vi "RTD_try_open.vi"(8 "error in":errorcluster, 11 "thermo in":T1={"type"=enum."COMET Tx5xx (ethernet)", "comment"="", "tag"="", "refresh"=0.0, "IP"="", "port"=0, "VISA"="", "last readout"=timestamp(0 s since 1904-01-01), "TCP ref"=refnum, "VISA sess"="", "idn"="", "press"=0.0, "RH"=0.0, "temp"=0.0, "pres cor"=[], "RH cor"=[], "temp cor"=[], "try left"=0, "failed"=FALSE, "RTD set"=[], "RTD inv"=[], "range"=0.0, "net mode"=enum."MODBUS", "try fail"=enum."Stop trying - return NaN", "timeout [s]"=0.0, "max retries"=0, "sim t [deg]"=0.0, "status"=0} {"status" items=["ok", "retry", "failed"]; "RTD inv" format="%.1f"; "RTD set" format="%.1f"; "temp cor" format="%.1f"; "RH cor" format="%.1f"; "pres cor" format="%.1f"; "refresh" min=0.1 max=1000.0 format="%.2f"}) -> (0 "error out":errorcluster, 3 "thermo out":T1={"type"=enum."COMET Tx5xx (ethernet)", "comment"="", "tag"="", "refresh"=5.0, "IP"="", "port"=502, "VISA"="", "last readout"=timestamp(0 s since 1904-01-01), "TCP ref"=refnum, "VISA sess"="", "idn"="", "press"=0.0, "RH"=0.0, "temp"=0.0, "pres cor"=[], "RH cor"=[], "temp cor"=[], "try left"=0, "failed"=FALSE, "RTD set"=[], "RTD inv"=[], "range"=0.0, "net mode"=enum."MODBUS", "try fail"=enum."Stop trying - return NaN", "timeout [s]"=0.0, "max retries"=0, "sim t [deg]"=0.0, "status"=0} {"status" items=["ok", "retry", "failed"]; "RTD inv" format="%.1f"; "RTD set" format="%.1f"; "temp cor" format="%.1f"; "RH cor" format="%.1f"; "pres cor" format="%.1f"; "refresh" min=0.1 max=1000.0 format="%.2f"})   [LabVIEW 2020]
uses:
  thermo.ctl
  thermo_types.ctl
  Thermometer Fail Action.ctl
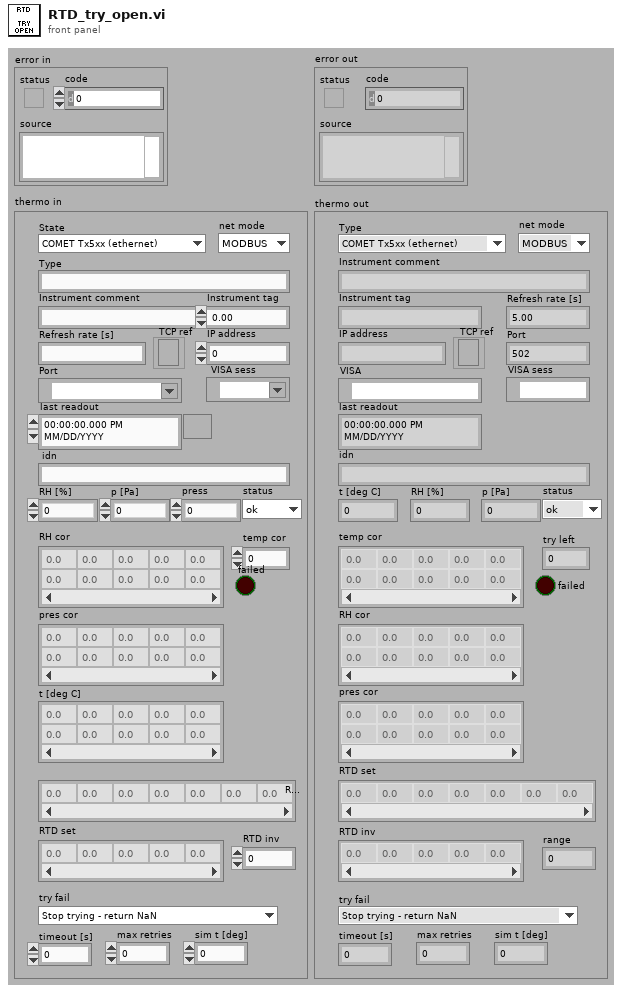
[diagram p1: front panel]
types:
  T1 = typedef "thermo.ctl" = cluster{"type":T2, "comment":string, "tag":string, "refresh":dbl, "IP":string, "port":u16, "VISA":refnum<visa-resource-name>, "last readout":timestamp, "TCP ref":refnum<k5>, "VISA sess":refnum<visa-resource-name>, "idn":string, "press":dbl, "RH":dbl, "temp":dbl, "pres cor":dbl[][], "RH cor":dbl[][], "temp cor":dbl[][], "try left":i32, "failed":bool, "RTD set":dbl[], "RTD inv":dbl[], "range":dbl, "net mode":enum16{"MODBUS", "HTTP"}, "try fail":T3, "timeout [s]":dbl, "max retries":i32, "sim t [deg]":dbl, "status":u16}
  T2 = typedef "thermo_types.ctl" = enum16{"Disabled", "Simulated", "COMET Tx5xx (ethernet)", "Keithley 2002 (GPIB) + RTD", "Agilent 344xx (GPIB) + RTD"}
  T3 = typedef "Thermometer Fail Action.ctl" = enum16{"Stop trying - keep last value", "Stop trying - return NaN", "Generate error - stop sweep"}
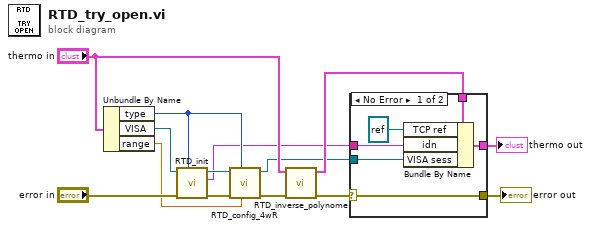
[diagram p0: block diagram]
diagram:
  n1 = Unbundle By Name("thermo in") -> ("type"=w9:T2, "VISA"=w10:refnum<visa-resource-name>, "range"=w8:dbl)
  n2 = call "RTD_init.vi"("type"=w9, "error in"="error in", "VISA in"=w10) -> ("error out"=w14:errorcluster, "ID"=w5:string, "VISA out"=w13:refnum<visa-resource-name>)  [unwired: 6 in]
  n3 = call "RTD_config_4wR.vi"("range [Ohm]"=w8, "type"=w9, "error in"=w14, "VISA in"=w13) -> ("error out"=w12:errorcluster, "VISA out"=w4:refnum<visa-resource-name>)  [unwired: 6 in]
  n4 = call "RTD_inverse_polynome.vi"("error in"=w12, "channel in"="thermo in") -> ("error out"=w3:errorcluster, "channel out"=w6:T1)  [unwired: 8 in]
  n5 = case shown="No Error" w3 {
    selector: w3 -> [w16 w22]
    tunnel: w6 -> [w20 w21]
    tunnel: w5 -> [w19 _]
    tunnel: w4 -> [w17 _]
    tunnel: [w16 w22] -> w2
    tunnel: [w15 w21] -> w1
    frame No Error {
      n6 = Bundle By Name(cluster=w20, "TCP ref"=refnum<k5> refnum, "idn"=w19, "VISA sess"=w17) -> (w15:T1)
    }
    frame Error {
    }
  }
  "error out" <- w2
  "thermo out" <- w1
